vi "User Interface Event Handler.vi"() -> ()   [LabVIEW 2020]
uses:
  <vilib>/DAQmx/create/channels.llb/DAQmx Create Channel (AI-Voltage-Basic).vi
  <vilib>/DAQmx/read.llb/DAQmx Read (Analog 2D DBL NChan NSamp).vi
  <vilib>/DAQmx/configure/timing.llb/DAQmx Timing (Sample Clock).vi
  <vilib>/Utility/file.llb/Write Delimited Spreadsheet (DBL).vi
  <vilib>/DAQmx/write.llb/DAQmx Write (Analog DBL 1Chan 1Samp).vi
  <vilib>/DAQmx/create/channels.llb/DAQmx Create Channel (AO-Voltage-Basic).vi
panel:
  in  "Generate Stimulus":bool
  in  "AO Voltage Channel":tag
  in  "Acquire":bool
  in  "Analyze":bool
  in  "Save Data":bool
  in  "Clear":bool
  in  "Exit":bool
  in  "Samples per channel":i32
  in  "Sample Rate":dbl
  in  "AI Voltage Channel":tag
  out "Graph":dbl[](graph)
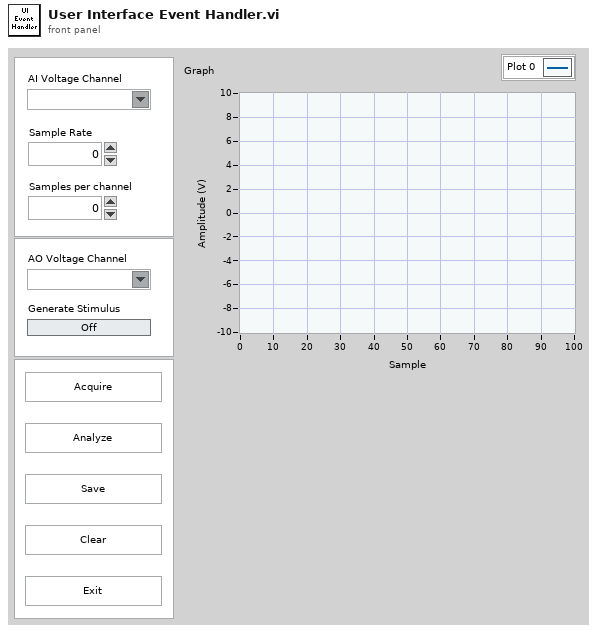
[diagram p1: front panel]
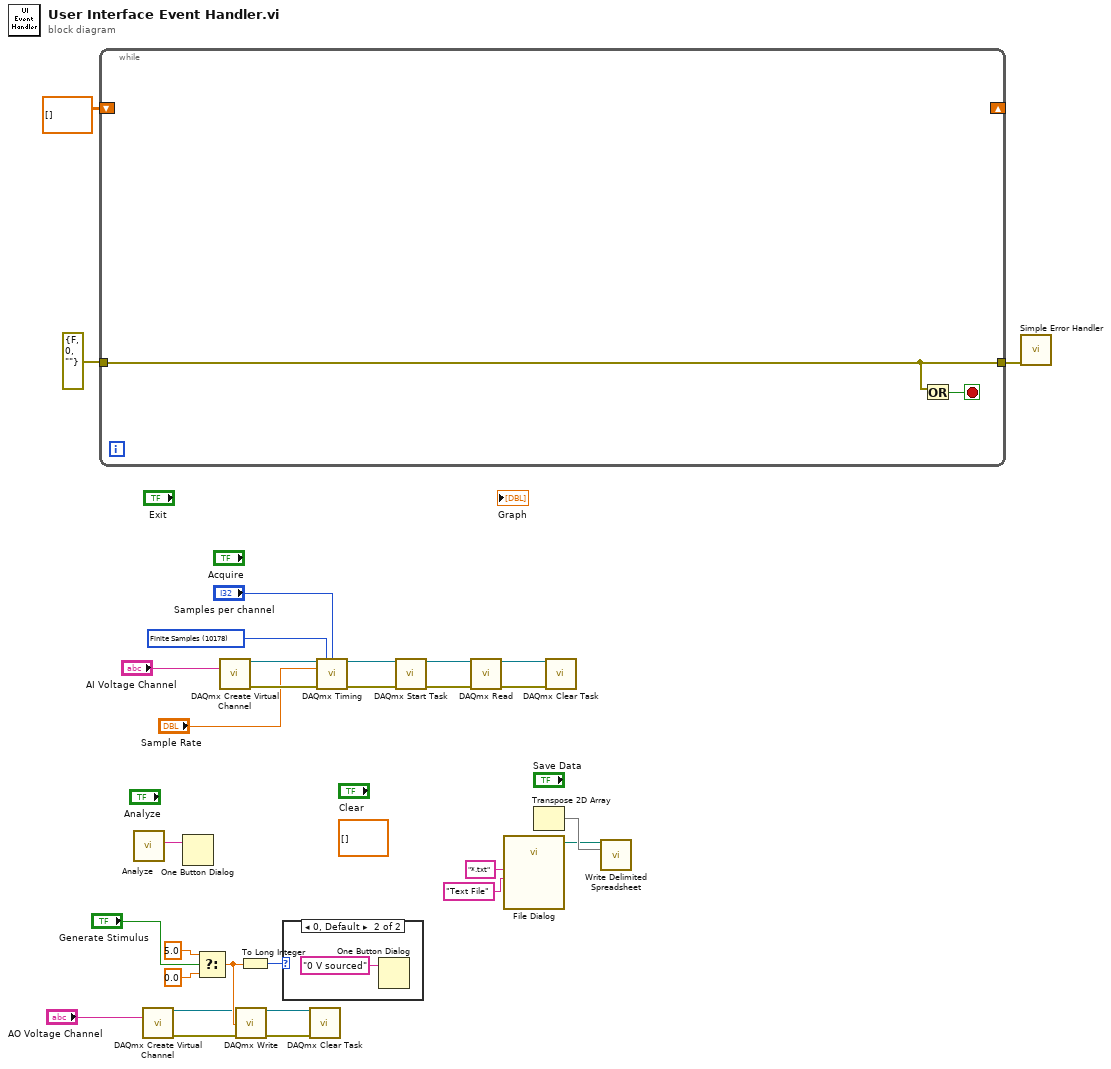
[diagram p0: block diagram]
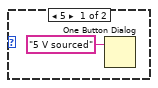
[diagram p2: hidden frame]
diagram:
  (unwired) dbl[][] []
  w18 = 10178 items=["Finite Samples"=10178, "Continuous Samples"=10123, "Hardware Timed Single Point"=12522] ("sample mode")
  n1 = while {
    shift-right: _ -> [_]
    shift-left: dbl[][] [] -> [_]
    tunnel: errorcluster {"status"=FALSE, "code"=0, "source"=""} ("error constant") -> [w32]
    tunnel: [w32] -> w30
    stop <- w31 stop-if-true
    n2 = Or(x=w32) -> (x .or. y?=w31:bool)  [unwired: 1 in]
  }
  n3 = call "Analyze.vi"() -> ("message"=w1:string)  [unwired: 8 in, 1 out]
  n4 = call-poly <vilib>:"DAQmx Create Virtual Channel.vi"("physical channels"="AO Voltage Channel") -> ("task out"=w5:refnum<k21>, "error out"=w4:errorcluster)  [unwired: 13 in]
  n5 = One Button Dialog(message=w1) -> ()  [unwired: 1 in, 1 out]
  n6 = Select(t=5.0, s="Generate Stimulus", f=0.0) -> (s? t:f=w9:dbl)
  n7 = call-poly <vilib>:"DAQmx Create Virtual Channel.vi"("physical channels"="AI Voltage Channel") -> ("task out"=w27:refnum<k21>, "error out"=w26:errorcluster)  [unwired: 13 in]
  n8 = call-poly <vilib>:"DAQmx Write.vi"("task/channels in"=w5, "data"=w9, "error in"=w4) -> ("task out"=w3:refnum<k21>, "error out"=w2:errorcluster)  [unwired: 10 in, 1 out]
  n9 = To Long Integer(number=w9) -> (32bit integer=w8:i32)
  n10 = case shown="0, Default" w8 {
    frame 5 {
      n11 = One Button Dialog(message="5 V sourced") -> ()  [unwired: 1 in, 1 out]
    }
    frame 0, Default {
      n12 = One Button Dialog(message="0 V sourced") -> ()  [unwired: 1 in, 1 out]
    }
  }
  n13 = call <vilib>:"DAQmx Clear Task.vi"("task in"=w3, "error in"=w2) -> ()  [unwired: 13 in, 1 out]
  n14 = call-poly <vilib>:"DAQmx Timing.vi"("task/channels in"=w27, "sample mode"=w18, "samples per channel"="Samples per channel", "rate"="Sample Rate", "error in"=w26) -> ("task out"=w25:refnum<k21>, "error out"=w24:errorcluster)  [unwired: 9 in]
  n15 = call <vilib>:"DAQmx Start Task.vi"("task/channels in"=w25, "error in"=w24) -> ("task out"=w23:refnum<k21>, "error out"=w22:errorcluster)  [unwired: 12 in]
  n16 = call-poly <vilib>:"DAQmx Read.vi"("task/channels in"=w23, "error in"=w22) -> ("task out"=w21:refnum<k21>, "error out"=w20:errorcluster)  [unwired: 11 in, 1 out]
  n17 = call "File Dialog"("pattern (all files)"="*.txt", "pattern label"="Text File") -> ("selected path"=w14:path)  [unwired: 10 in, 3 out]
  n18 = Transpose 2D Array() -> (transposed array=w15:dbl[][])  [unwired: 1 in]
  n19 = call <vilib>:"DAQmx Clear Task.vi"("task in"=w21, "error in"=w20) -> ()  [unwired: 13 in, 1 out]
  n20 = call-poly <vilib>:"Write Delimited Spreadsheet.vi"("file path (dialog if empty)"=w14, "2D data"=w15) -> ()  [unwired: 12 in, 2 out]
  n21 = call <vilib>:"Simple Error Handler.vi"("error in (no error)"=w30) -> ()  [unwired: 4 in, 5 out]
